vi "Newmark-Initializa.vi"() -> ()   [LabVIEW 2011]
uses:
  <vilib>/Instr/_visa.llb/VISA Configure Serial Port (Instr).vi
panel:
  out "Communication Log":string
  in  "Timeout":u32=10000
  in  "baud rate":u32=9600
  in  "VISA resource name":refnum<visa-resource-name>
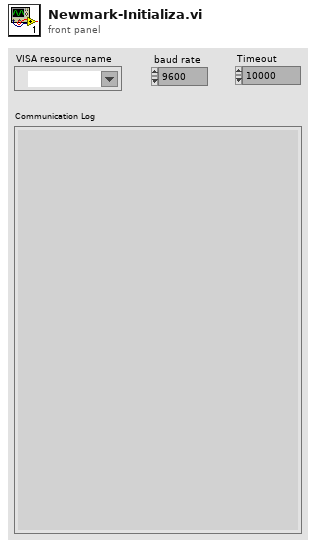
[diagram p1: front panel]
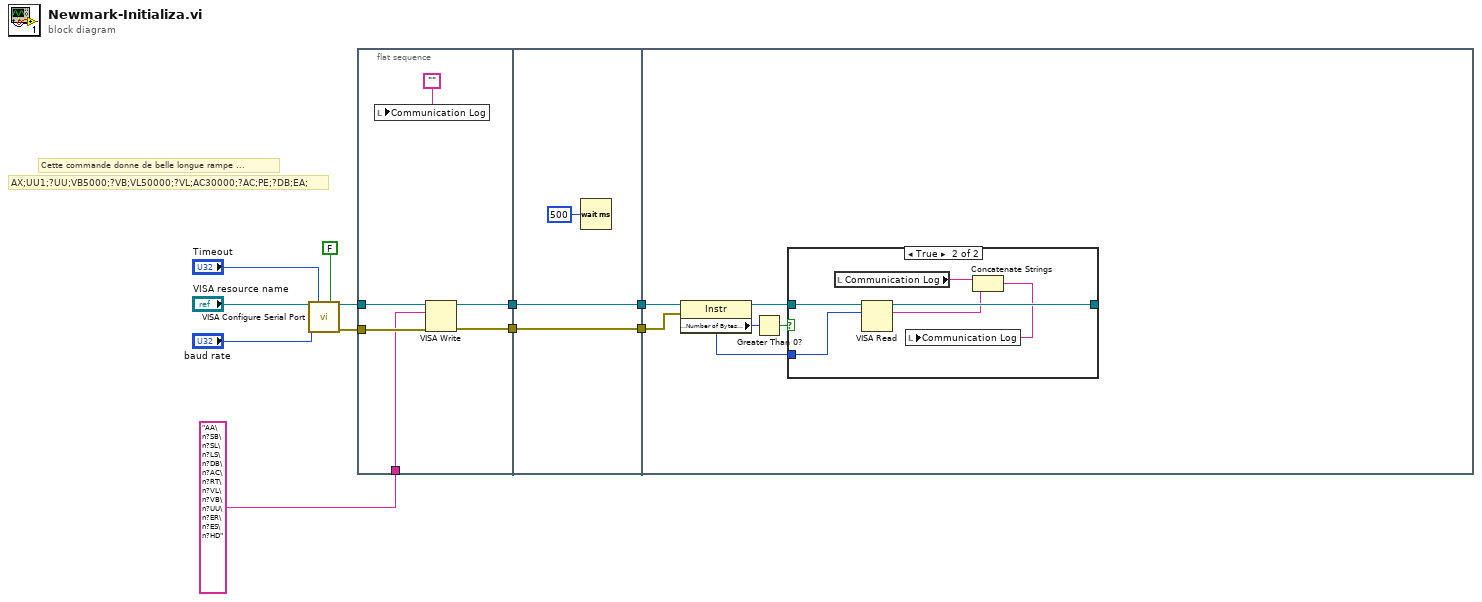
[diagram p0: block diagram]
diagram:
  # "Cette commande donne de belle longue rampe ..."
  # "AX;UU1;?UU;VB5000;?VB;VL50000;?VL;AC30000;?AC;PE;?DB;EA;"
  n1 = call-poly "VISA Configure Serial Port"("VISA resource name"="VISA resource name", "timeout (10sec)"="Timeout", "Enable Termination\nChar (T)"=FALSE ("Enable Termination\nChar (T)"), "baud rate (9600)"="baud rate") -> ("VISA resource name out"=w7:refnum<visa-resource-name>, "error out"=w6:errorcluster)  [unwired: 10 in]
  n2 = flat-sequence {
    tunnel: w7 -> [w17]
    tunnel: w6 -> [w16]
    tunnel: "AA\n?SB\n?SL\n?LS\n?DB\n?AC\n?RT\n?VL\n?VB\n?UU\n?ER\n?ES\n?HD" -> [w15]
    tunnel: [w14] -> w2
    tunnel: [w13] -> w4
    tunnel: w4 -> [w20]
    tunnel: [w20] -> w3
    tunnel: w2 -> [w19]
    tunnel: [w19] -> w1
    tunnel: w3 -> [w22]
    tunnel: w1 -> [w21]
    frame #0 {
      n3 = local write "Communication Log"("") -> ()
      n4 = VISA Write(VISA resource name=w17, write buffer=w15, error in (no error)=w16) -> (VISA resource name out=w13:refnum<visa-resource-name>, error out=w14:errorcluster)  [unwired: 1 out]
    }
    frame #1 {
      n5 = Wait (ms)(milliseconds to wait=u32 500) -> ()  [unwired: 1 out]
    }
    frame #2 {
      n6 = property class="Instr"(reference=w22, error in=w21) -> (reference out=w24:refnum<visa-resource-name>, "Serial Settings:Number of Bytes at Serial Port"=w25:u32)  [unwired: 1 out]
      n7 = Greater Than 0?(x=w25) -> (x > 0?=w23:bool)
      n8 = case shown="True" w23 {
        tunnel: w24 -> [w26 w32]
        tunnel: [w26 w30] -> _
        tunnel: w25 -> [_ w31]
        frame False {
        }
        frame True {
          n9 = local read "Communication Log"() -> (w28:string)
          n10 = VISA Read(VISA resource name=w32, byte count=w31) -> (VISA resource name out=w30:refnum<visa-resource-name>, read buffer=w29:string)  [unwired: 1 in, 2 out]
          n11 = Concatenate Strings(w28, w29) -> (w27:string)
          n12 = local write "Communication Log"(w27) -> ()
        }
      }
    }
  }
